vi "Average All.vi"(7 "Averaging":bool, 10 "Measurements":T1[](array[typedef])) -> (0 "Cart Forces":dbl[][](array[numeric]), 1 "Cart Disp":dbl[][](array[numeric]), 2 "Act Forces":dbl[][](array[numeric]), 3 "Act Disp":dbl[][](array[numeric]))   [LabVIEW 2009]
uses:
  Act & Cart Measurments.ctl
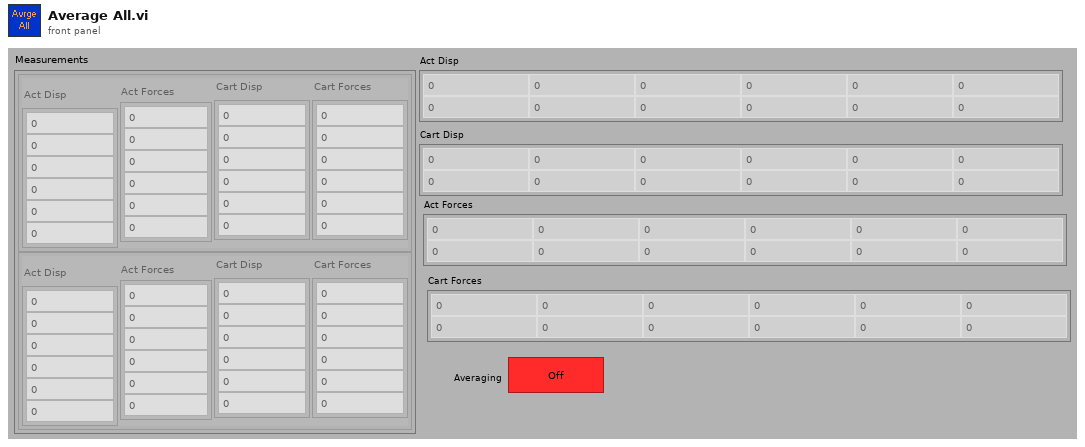
[diagram p1: front panel]
types:
  T1 = typedef "Act & Cart Measurments.ctl" = cluster{"Act Disp":dbl[], "Act Forces":dbl[], "Cart Disp":dbl[], "Cart Forces":dbl[]}
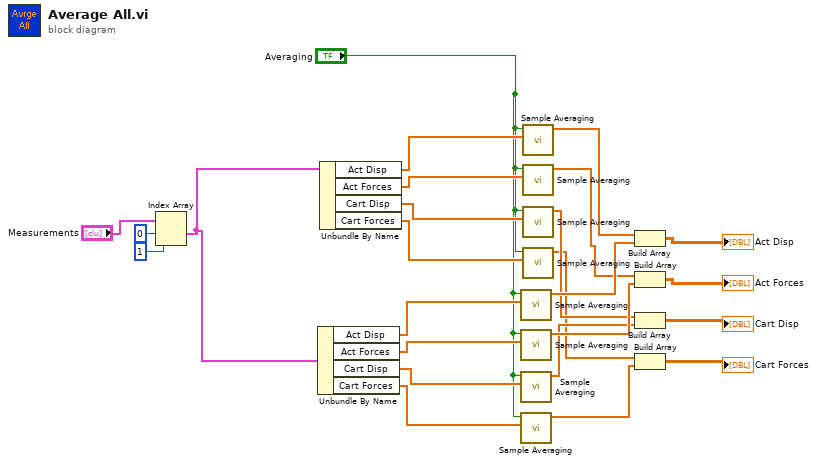
[diagram p0: block diagram]
diagram:
  n1 = Index Array(array="Measurements", index #1=0 ("index"), index #2=1 ("index")) -> (element #1=w13:T1)  [unwired: 1 out]
  n2 = Unbundle By Name(w13) -> ("Act Disp"=w21:dbl[], "Act Forces"=w20:dbl[], "Cart Disp"=w19:dbl[], "Cart Forces"=w18:dbl[])
  n3 = Unbundle By Name(w13) -> ("Act Disp"=w25:dbl[], "Act Forces"=w24:dbl[], "Cart Disp"=w23:dbl[], "Cart Forces"=w22:dbl[])
  n4 = call "Sample Averaging.vi"("Sample In"=w21, "Averaging"="Averaging") -> ("Sample Out"=w11:dbl[])  [unwired: 9 out]
  n5 = call "Sample Averaging.vi"("Sample In"=w20, "Averaging"="Averaging") -> ("Sample Out"=w9:dbl[])  [unwired: 9 out]
  n6 = call "Sample Averaging.vi"("Sample In"=w19, "Averaging"="Averaging") -> ("Sample Out"=w7:dbl[])  [unwired: 9 out]
  n7 = call "Sample Averaging.vi"("Sample In"=w18, "Averaging"="Averaging") -> ("Sample Out"=w5:dbl[])  [unwired: 9 out]
  n8 = call "Sample Averaging.vi"("Sample In"=w25, "Averaging"="Averaging") -> ("Sample Out"=w12:dbl[])  [unwired: 9 out]
  n9 = call "Sample Averaging.vi"("Sample In"=w24, "Averaging"="Averaging") -> ("Sample Out"=w10:dbl[])  [unwired: 9 out]
  n10 = call "Sample Averaging.vi"("Sample In"=w23, "Averaging"="Averaging") -> ("Sample Out"=w8:dbl[])  [unwired: 9 out]
  n11 = call "Sample Averaging.vi"("Sample In"=w22, "Averaging"="Averaging") -> ("Sample Out"=w6:dbl[])  [unwired: 9 out]
  n12 = Build Array(w12, w11) -> (→"Act Disp":dbl[][])
  n13 = Build Array(w10, w9) -> (→"Act Forces":dbl[][])
  n14 = Build Array(w8, w7) -> (→"Cart Disp":dbl[][])
  n15 = Build Array(w6, w5) -> (→"Cart Forces":dbl[][])
